vi "ECall.vi"(6 "error in (no error)":errorcluster, 9 "ECall":string[][](table)) -> (0 "error out":errorcluster, 3 "ECall":string[][](table))   [LabVIEW 2021]
panel:
  in  "Close":bool
  # "ECall"
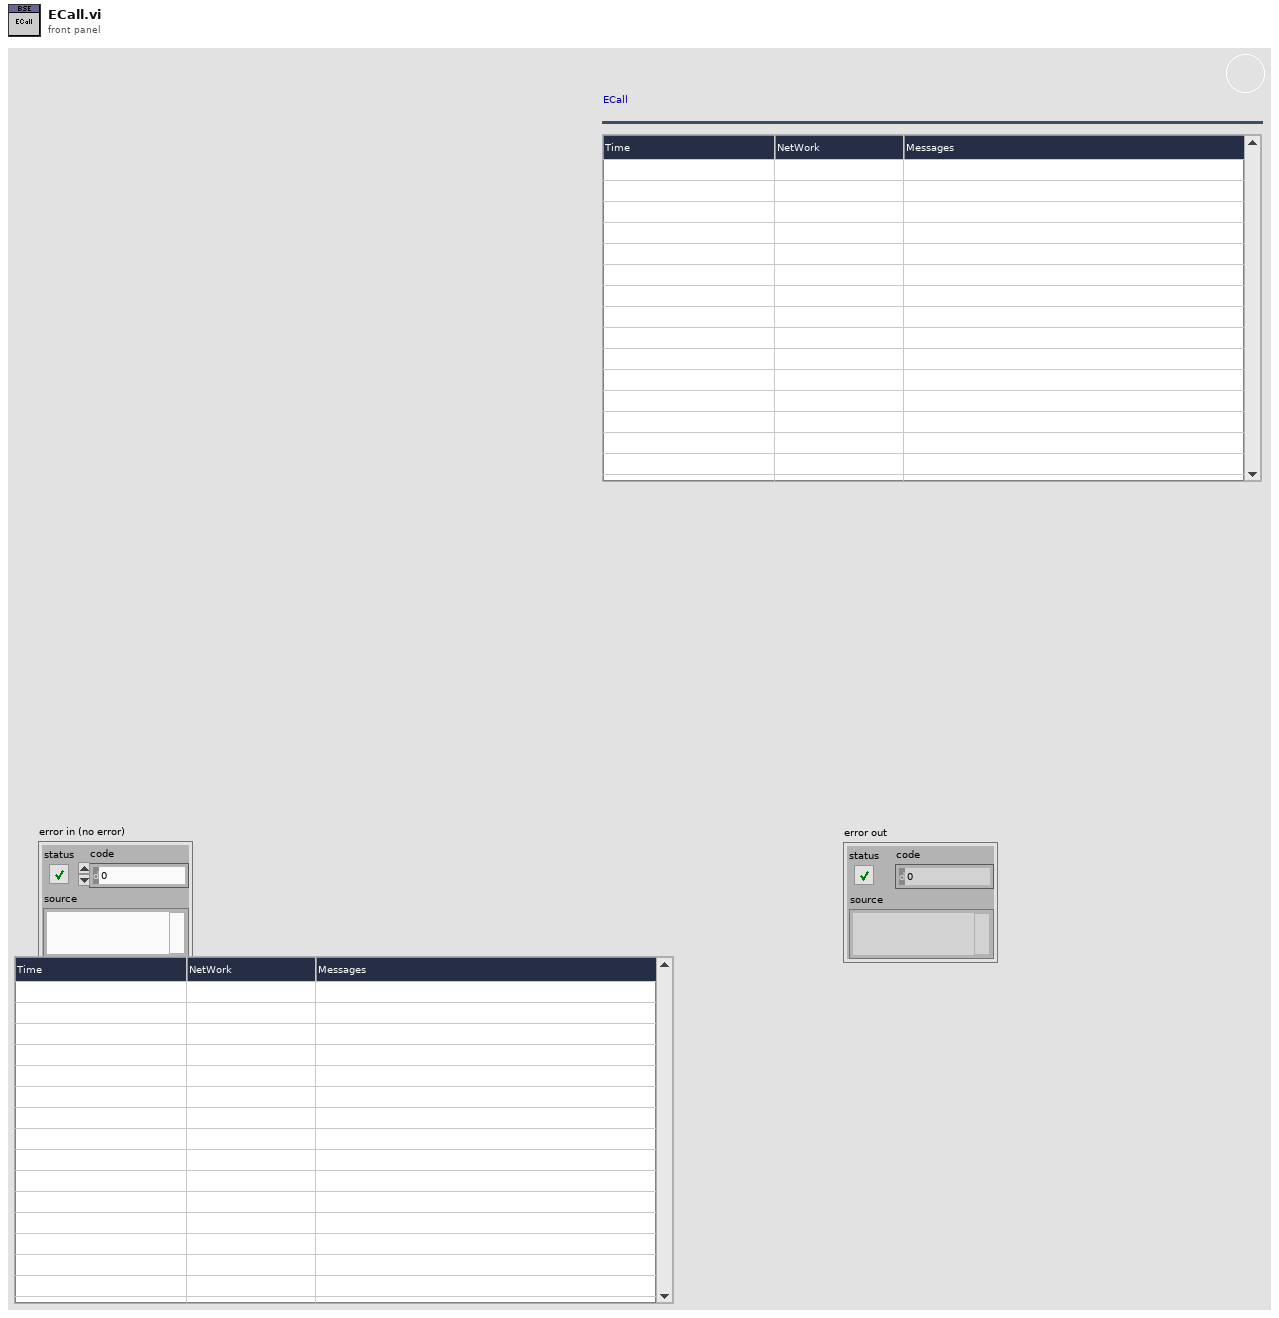
[diagram p1: front panel]
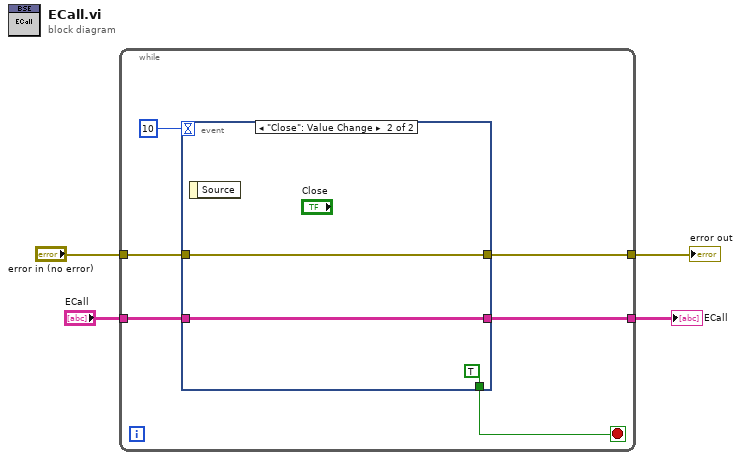
[diagram p0: block diagram]
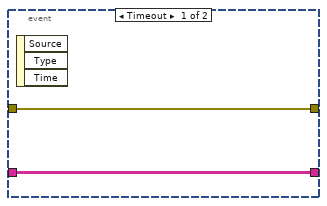
[diagram p2: hidden frame]
diagram:
  n1 = while {
    tunnel: "error in (no error)" -> [w8]
    tunnel: [w7] -> w3
    tunnel: "ECall" -> [w6]
    tunnel: [w5] -> w1
    stop <- w9 stop-if-true
    n2 = event shown="[1] \"Close\": Value Change" {
      selector: _ -> [_ _]
      dyn-events: _ -> [_ _]
      timeout: 10 -> [_ _]
      tunnel: [_ TRUE] -> w9
      tunnel: w8 -> [w12 w14]
      tunnel: [w12 w14] -> w7
      tunnel: w6 -> [w11 w13]
      tunnel: [w11 w13] -> w5
      event Timeout {
        n3 = event-data() -> ()  [unwired: 1 in, 3 out]
      }
      event "Close": Value Change {
        n4 = event-data() -> ()  [unwired: 1 in, 1 out]
      }
    }
  }
  "error out" <- w3
  "ECall" <- w1
